vi "3Axis_Rate_v2.vi"(9 "Roll_R":dbl, 10 "Yaw_R":dbl, 11 "Pitch_R":dbl) -> (0 "RRH":u8, 1 "YRL":u8, 2 "YRH":u8, 3 "PRL":u8, 4 "RRL":u8, 5 "PRH":u8)   [LabVIEW 2017]
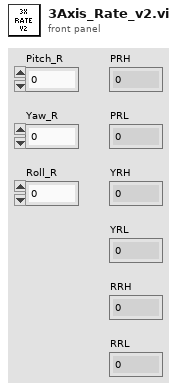
[diagram p1: front panel]
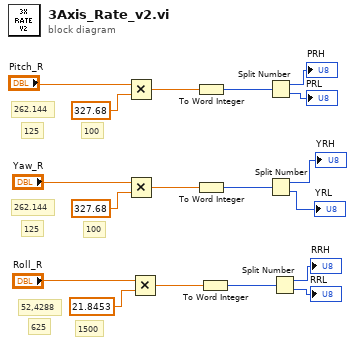
[diagram p0: block diagram]
diagram:
  # "625"
  # "52,4288"
  # "100"
  # "262.144"
  # "125"
  # "100"
  # "262.144"
  # "125"
  # "1500"
  n1 = Multiply(x="Pitch_R", y=327.68) -> (x*y=w7:dbl)
  n2 = Multiply(x="Yaw_R", y=327.68) -> (x*y=w3:dbl)
  n3 = Multiply(x="Roll_R", y=21.8453) -> (x*y=w10:dbl)
  n4 = To Word Integer(number=w7) -> (16bit integer=w5:i16)
  n5 = To Word Integer(number=w3) -> (16bit integer=w4:i16)
  n6 = To Word Integer(number=w10) -> (16bit integer=w6:i16)
  n7 = Split Number(x=w5) -> (hi(x)=→"PRH":u8, lo(x)=→"PRL":u8)
  n8 = Split Number(x=w4) -> (hi(x)=→"YRH":u8, lo(x)=→"YRL":u8)
  n9 = Split Number(x=w6) -> (hi(x)=→"RRH":u8, lo(x)=→"RRL":u8)
